vi "Get 1D Unique.vi"(2 "Array":u64[](array[numeric])) -> (14 "unique":u64[](array[numeric]), 16 "index lookup":i64[](array[numeric]), 17 "count":u64, 18 "max":u64, 19 "min":u64)   [LabVIEW 2014]
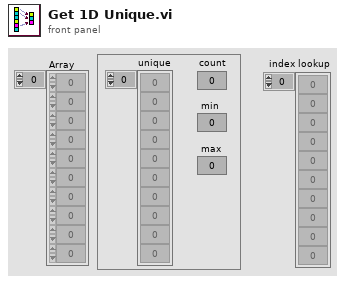
[diagram p1: front panel]
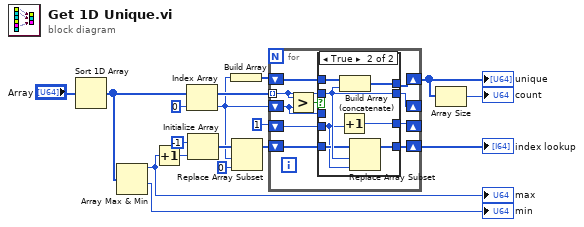
[diagram p0: block diagram]
diagram:
  n1 = Sort 1D Array(array="Array") -> (sorted array=w10:u64[])
  n2 = Array Max & Min(array=w10) -> (max value=w9:u64, min value=→"min":u64)  [unwired: 2 out]
  "max" <- w9
  n3 = Increment(x=w9) -> (x+1=w8:u64)
  n4 = Index Array(array=w10, index=0) -> (element=w3:u64)
  n5 = Initialize Array(i64 -1 ("element"), w8) -> (w5:i64[])
  n6 = Build Array(w3) -> (w14:u64[])
  n7 = Replace Array Subset(array=w5, new element=0 ("index"), index=w3) -> (w4:i64[])
  n8 = for {
    tunnel: w10 -> [w24] mode=indexing
    shift-right: [w23] -> _
    shift-left: w3 -> [w25]
    shift-right: [w22] -> w13
    shift-left: w14 -> [w21]
    shift-right: [w19] -> w1
    shift-left: w4 -> [w20]
    shift-right: [w17] -> _
    shift-left: 1 ("index") -> [w18]
    n9 = Greater?(x=w24, y=w25) -> (0:w26:bool)
    n10 = case shown="True" w26 {
      tunnel: w25 -> [w30 _]
      tunnel: w24 -> [_ w35]
      tunnel: [w30 w35] -> w23
      tunnel: [w29 w37] -> w22
      tunnel: w21 -> [w29 w36]
      tunnel: w20 -> [w27 w34]
      tunnel: [w27 w33] -> w19
      tunnel: w18 -> [w28 w32]
      tunnel: [w28 w31] -> w17
      frame False {
      }
      frame True {
        n11 = Increment(x=w32) -> (x+1=w31:i32)
        n12 = Build Array (concatenate)(w36, w35) -> (w37:u64[])
        n13 = Replace Array Subset(array=w34, new element=w32, index=w35) -> (w33:i64[])
      }
    }
  }
  "unique" <- w13
  "index lookup" <- w1
  n14 = Array Size(array=w13) -> (size(s)=→"count":i32)
